vi "calculate_value_tolerance_by_equal.vi"(10 "measured_value":dbl[][](array[numeric]), 11 "tolerance_list":T1) -> (3 "Array":cluster{"MIN":dbl, "MAX":dbl}[][](array[cluster]))   [LabVIEW 2017]
uses:
  types/tolerance_list.ctl
  types/tolerance.ctl
panel:
  out "error out":errorcluster
  in  "error in (no error)":errorcluster
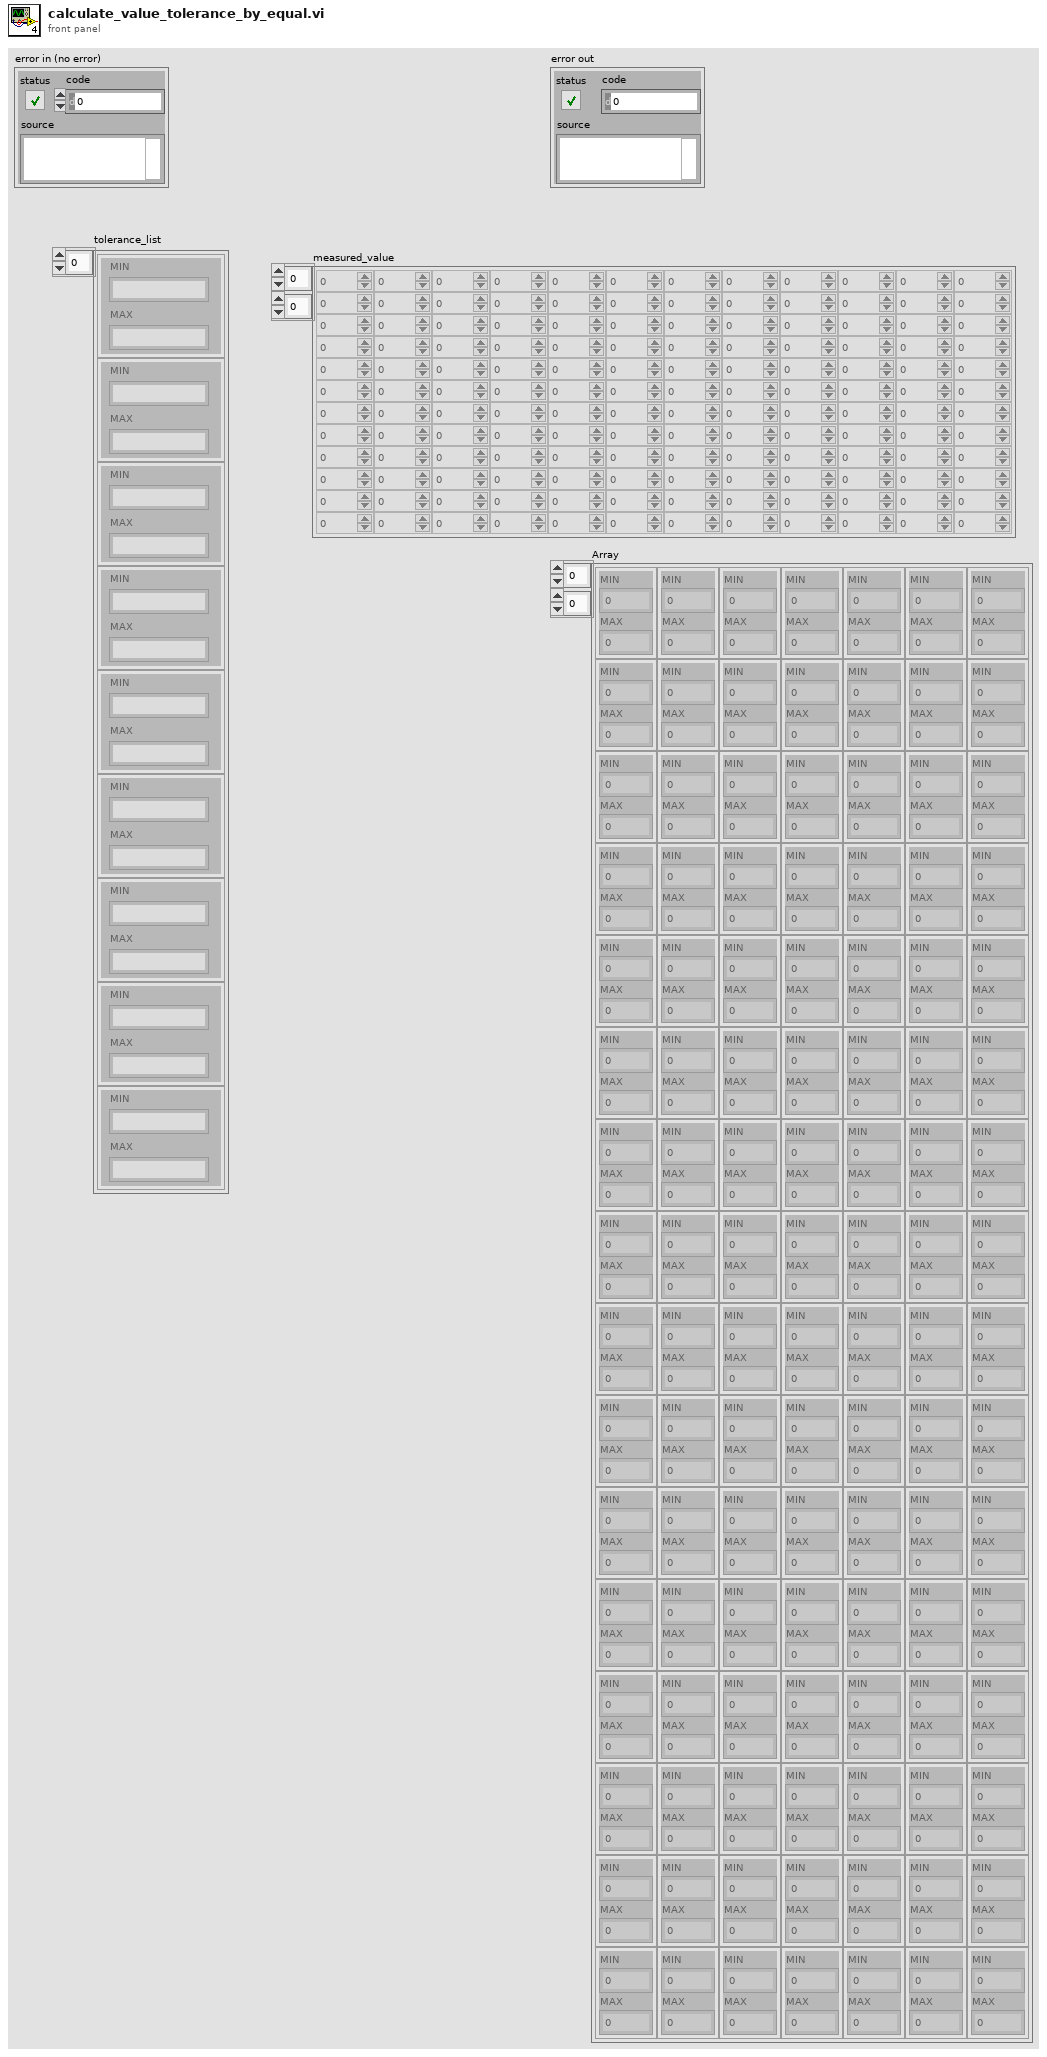
[diagram p1: front panel]
types:
  T1 = typedef "tolerance_list.ctl" = T2[]
  T2 = typedef "tolerance.ctl" = cluster{"MIN":string, "MAX":string}
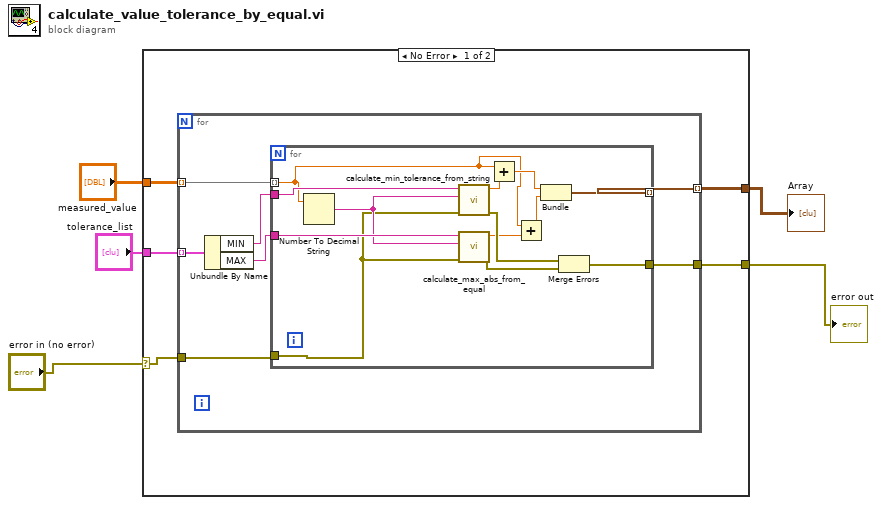
[diagram p0: block diagram]
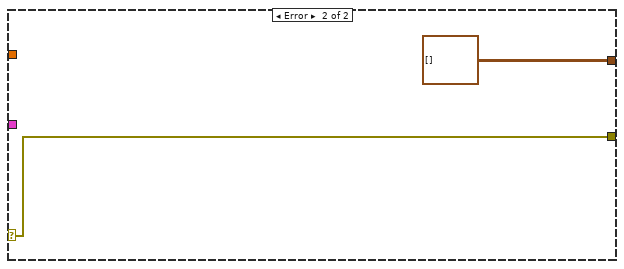
[diagram p2: hidden frame]
diagram:
  n1 = case shown="No Error" "error in (no error)" {
    selector: "error in (no error)" -> [w7 w32]
    tunnel: "tolerance_list" -> [w10 _]
    tunnel: "measured_value" -> [w9 _]
    tunnel: [w8 cluster{"MIN":dbl, "MAX":dbl}[][] []] -> w3
    tunnel: [w6 w32] -> w1
    frame No Error {
      n2 = for {
        tunnel: w10 -> [w17] mode=indexing
        tunnel: w9 -> [w16] mode=indexing
        tunnel: [w13] -> w8 mode=indexing
        tunnel: w7 -> [w12]
        tunnel: [w11] -> w6
        n3 = Unbundle By Name(w17) -> ("MIN"=w15:string, "MAX"=w14:string)
        n4 = for {
          tunnel: w16 -> [w19] mode=indexing
          tunnel: w15 -> [w30]
          tunnel: w14 -> [w29]
          tunnel: [w27] -> w13 mode=indexing
          tunnel: w12 -> [w24]
          tunnel: [w23] -> w11
          n5 = Number To Decimal String(number=w19) -> (decimal integer string=w28:string)  [unwired: 1 in]
          n6 = call "calculate_min_tolerance_from_string.vi"("error in (no error)"=w24, "String"=w28, "MIN"=w30) -> ("error out"=w26:errorcluster, "MIN"=w22:dbl)  [unwired: 7 in]
          n7 = call "calculate_max_abs_from_equal.vi"("error in (no error)"=w24, "String"=w28, "MAX"=w29) -> ("error out"=w25:errorcluster, "MAX"=w20:dbl)  [unwired: 7 in]
          n8 = Add(x=w19, y=w22) -> (x+y=w21:dbl)
          n9 = Add(x=w19, y=w20) -> (x+y=w18:dbl)
          n10 = Bundle(w21, w18) -> (w27:cluster{dbl, dbl})  [unwired: 1 in]
          n11 = Merge Errors(w26, w25) -> (w23:errorcluster)
        }
      }
    }
    frame Error {
    }
  }
  "Array" <- w3
  "error out" <- w1
